vi "Main_SubVI_Hex to Result Array.vi"(8 "Error In":errorcluster, 11 "Hex In":string) -> (0 "Error Out":errorcluster, 3 "Normal Array Out":string[](array[string]))   [LabVIEW 2015]
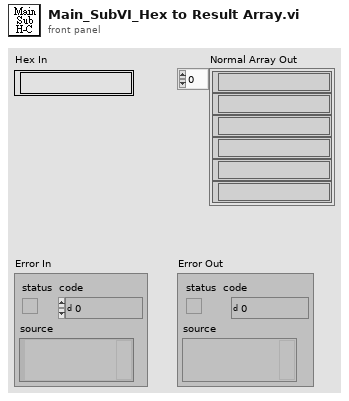
[diagram p1: front panel]
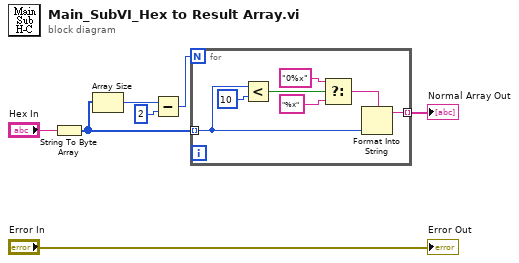
[diagram p0: block diagram]
diagram:
  n1 = String To Byte Array(string="Hex In") -> (unsigned byte array=w4:u8[])
  n2 = Array Size(array=w4) -> (size(s)=w6:i32)
  n3 = Subtract(x=w6, y=2) -> (x-y=w5:i32)
  n4 = for {
    N: w5 -> [_]
    tunnel: w4 -> [w9] mode=indexing
    tunnel: [w8] -> w3 mode=indexing
    n5 = Less?(x=w9, y=u8 10) -> (x < y?=w13:bool)
    n6 = Select(t="0%x", s=w13, f="%x") -> (s? t:f=w12:string)
    n7 = Format Into String(format string=w12, w9) -> (resulting string=w8:string)  [unwired: 2 in, 1 out]
  }
  "Normal Array Out" <- w3
  "Error Out" <- "Error In"
